vi "FTW-Actor-GetNextJob.vi"(8 "error in":errorcluster, 10 "Jobs Performed":i32, 11 "FTW Actor Instance":refnum<class "FTW-ActorInstance.lvclass">) -> (0 "error out":errorcluster, 1 "Job Data":string, 2 "Job Name":string, 3 "FTW Actor Instance out":refnum<class "FTW-ActorInstance.lvclass">)   [LabVIEW 2012, in "FTW-Actor.lvlib" / "FTW-ActorInstance.lvclass"]
uses:
  FTW-ActorInstance.lvclass
  FTW-ActorInstance.lvclass/FTW-ActorInstance.ctl
  JobSequencer/FTW-JobSequencer.lvclass
panel:
  # "Inputs"
  # "Outputs"
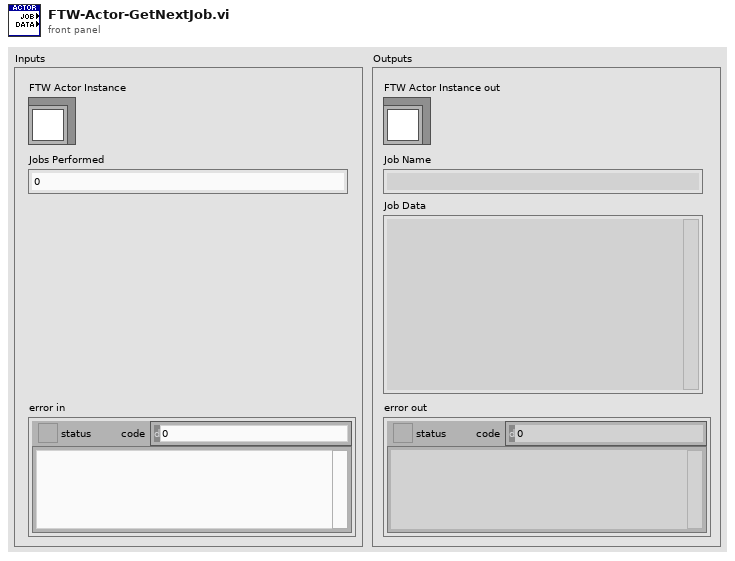
[diagram p1: front panel]
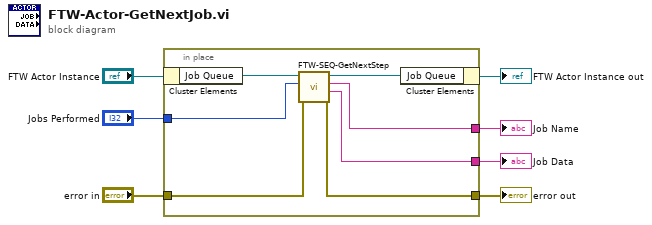
[diagram p0: block diagram]
diagram:
  n1 = in-place {
    in-place-border: "error in" -> [w14]
    in-place-border: [w13] -> w6
    in-place-border: [w10] -> w4
    in-place-border: [w9] -> w3
    in-place-border: "Jobs Performed" -> [w8]
    n2 = in-place-cluster #1("FTW Actor Instance") -> ("Job Queue"=w12:refnum<class "FTW-JobSequencer.lvclass">)
    n3 = call "FTW-SEQ-GetNextStep.vi"("error in"=w14, "Jobs Performed"=w8, "FTW Job Sequencer"=w12) -> ("error out"=w13:errorcluster, "Job Data"=w9:string, "Current Job"=w10:string, "FTW Job Sequencer out"=w11:refnum<class "FTW-JobSequencer.lvclass">)  [unwired: 5 in]
    n4 = in-place-cluster #1("Job Queue"=w11) -> (→"FTW Actor Instance out":refnum<class "FTW-ActorInstance.lvclass">)
  }
  "error out" <- w6
  "Job Name" <- w4
  "Job Data" <- w3
